vi "TL calculate steering angle.vi"(1 "Compass\nheading":dbl format="%#_13g", 2 "New heading":dbl format="%#_13g") -> (0 "Local Steering Angle":dbl)   [LabVIEW 2014]
doc: "This VI calculates a steering angle in the local coordinates based upon the present compass heading and a desired new heading."
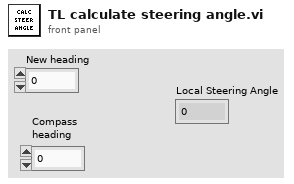
[diagram p1: front panel]
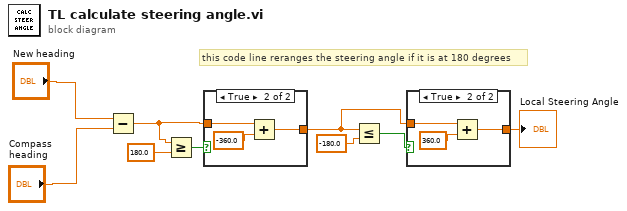
[diagram p0: block diagram]
diagram:
  # "this code line reranges the steering angle if it is at 180 degrees"
  n1 = Subtract(x="New heading", y="Compass\nheading") -> (x-y=w2:dbl)
  n2 = Greater Or Equal?(x=w2, y=180.0) -> (x >= y?=w8:bool)
  n3 = case shown="True" w8 {
    tunnel: w2 -> [w10 w13]
    tunnel: [w10 w11] -> w5
    frame False {
    }
    frame True {
      n4 = Add(x=w13, y=-360.0) -> (x+y=w11:dbl)
    }
  }
  n5 = Less Or Equal?(x=w5, y=-180.0) -> (x <= y?=w6:bool)
  n6 = case shown="True" w6 {
    tunnel: w5 -> [w14 w17]
    tunnel: [w14 w15] -> w1
    frame False {
    }
    frame True {
      n7 = Add(x=w17, y=360.0) -> (x+y=w15:dbl)
    }
  }
  "Local Steering Angle" <- w1
